vi "ServiceSendBytesRoutedMessage_Create.vi"(7 "Header":T2, 8 "error in (no error)":errorcluster, 10 "SendTo":string, 11 "ServiceSendBytesRoutedMessage":T1) -> (0 "error out":errorcluster, 3 "Message":T4)   [LabVIEW 2017]
uses:
  <vilib>/addons/InsightCM/MessageBus/Base/controls/Message.ctl
  <vilib>/addons/InsightCM/MessageBus/Base/controls/MessageHeader.ctl
  <vilib>/addons/InsightCM/MessageBus/Base/controls/KeyValuePair.ctl
  <vilib>/addons/InsightCM/MessageBus/MessageLibrary/Service/controls/ServiceSendBytesRoutedMessageBody.ctl
  <vilib>/addons/InsightCM/MessageBus/Base/controls/MessageClassType.ctl
  <vilib>/addons/InsightCM/Utilities/PropertyHelpers/PropertyHelpers.lvlib
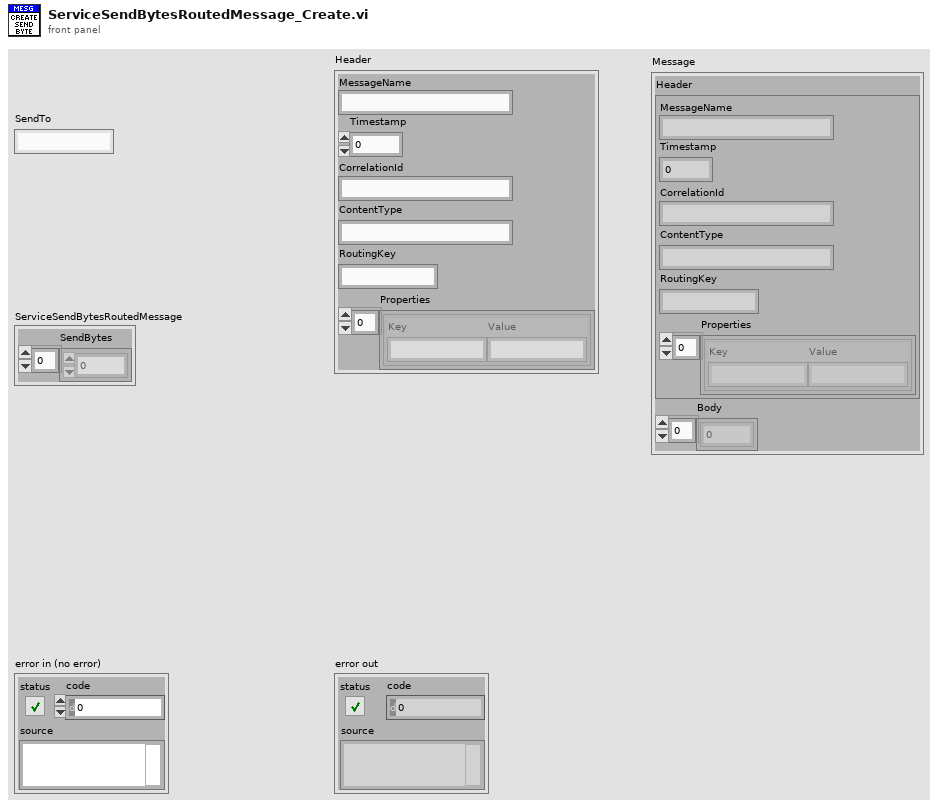
[diagram p1: front panel]
types:
  T1 = typedef "ServiceSendBytesRoutedMessageBody.ctl" = cluster{"SendBytes":u8[]}
  T2 = typedef "MessageHeader.ctl" = cluster{"MessageName":string, "Timestamp":i64, "CorrelationId":string, "ContentType":string, "RoutingKey":string, "Properties":T3[]}
  T3 = typedef "KeyValuePair.ctl" = cluster{"Key":string, "Value":string}
  T4 = typedef "Message.ctl" = cluster{"Header":T2, "Body":u8[]}
  T5 = typedef "MessageClassType.ctl" = enum16{"Request", "Response", "Broadcast", "RoutedMessage"}
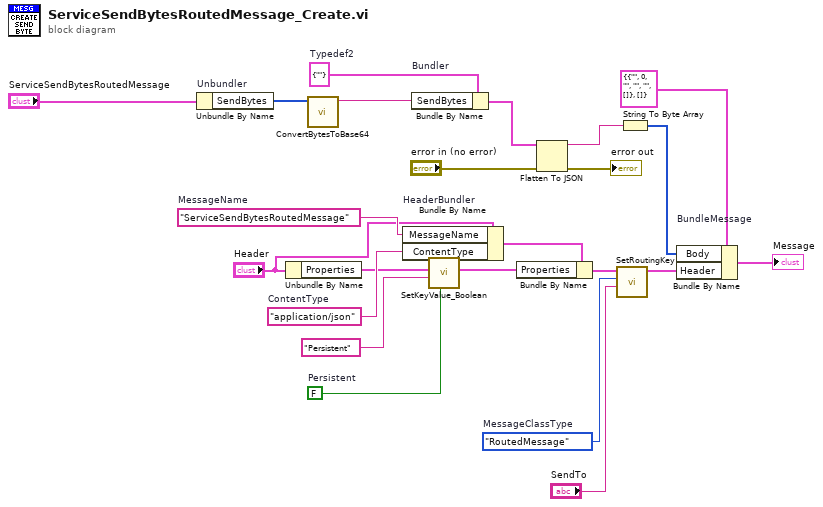
[diagram p0: block diagram]
diagram:
  w3 = cluster{"SendBytes":string} {"SendBytes"=""}  # Typedef2
  w19 = MessageClassType."RoutedMessage"  # MessageClassType
  w14 = FALSE  # Persistent
  w20 = "ServiceSendBytesRoutedMessage"  # MessageName
  w17 = "application/json"  # ContentType
  n1 = Unbundle By Name "Unbundler"("ServiceSendBytesRoutedMessage") -> ("SendBytes"=w2:u8[])
  n2 = Unbundle By Name("Header") -> ("Properties"=w16:T3[])
  n3 = call <vilib>:"ConvertBytesToBase64.vi"("U8 array"=w2) -> ("base64 encoded"=w1:string)  [unwired: 10 in]
  n4 = Bundle By Name "HeaderBundler"(cluster="Header", "MessageName"=w20, "ContentType"=w17) -> (w11:T2)
  n5 = Bundle By Name "Bundler"(cluster=w3, "SendBytes"=w1) -> (w4:cluster{"SendBytes":string})
  n6 = call <vilib>:"SetKeyValue_Boolean.vi"("value"=w14, "key"="Persistent" ("Key"), "key value pairs"=w16) -> ("key value pairs out"=w10:T3[])  [unwired: 8 in]
  n7 = Bundle By Name(cluster=w11, "Properties"=w10) -> (w12:T2)
  n8 = Flatten To JSON(anything=w4, error in (no error)="error in (no error)") -> (JSON string=w6:string, 11:→"error out":errorcluster)  [unwired: 1 in]
  n9 = call <vilib>:"SetRoutingKey.vi"("SendTo"="SendTo", "MessageClassType"=w19, "Message Header in"=w12) -> ("Message Header out"=w13:T2)  [unwired: 8 in]
  n10 = String To Byte Array(string=w6) -> (unsigned byte array=w22:u8[])
  n11 = Bundle By Name "BundleMessage"(cluster=T4 {"Header"={"MessageName"="", "Timestamp"=0, "CorrelationId"="", "ContentType"="", "RoutingKey"="", "Properties"=[]}, "Body"=[]} ("Message"), "Body"=w22, "Header"=w13) -> (→"Message":T4)
